vi "PreK12Login.vi"(2 "error in (no error)":errorcluster, 3 "Admin?":bool) -> (0 "error out":errorcluster, 1 "connection ID out":refnum<k5>)   [LabVIEW 2012]
uses:
  <userlib>/BotSpeak/Devices/EvalRIO/FTPCodes/FTPGlobals.vi
panel:
  out "passwrd":bool
  out "user":bool
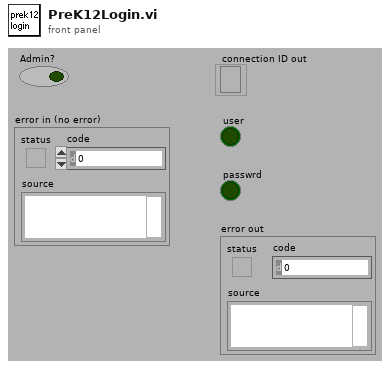
[diagram p1: front panel]
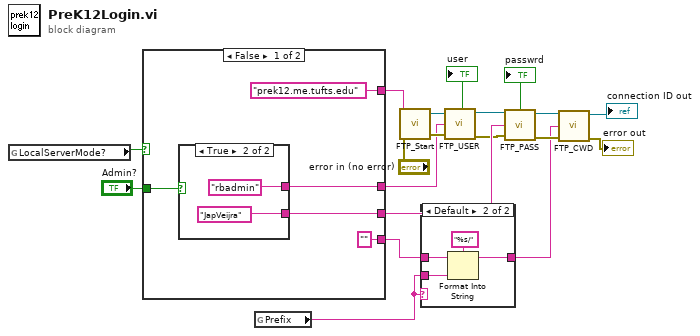
[diagram p0: block diagram]
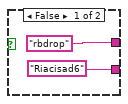
[diagram p3: hidden frame]
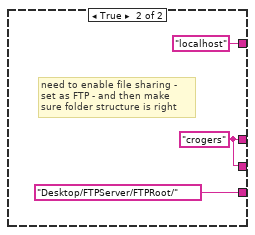
[diagram p4: hidden frame]
diagram:
  n1 = global read "FTPGlobals.vi" "LocalServerMode?"() -> (w2:bool)
  n2 = case shown="False" w2 {
    tunnel: [w24 w29] -> w14
    tunnel: [w23 w29] -> w13
    tunnel: "Admin?" -> [w22 _]
    tunnel: ["prek12.me.tufts.edu" ("address") "localhost" ("address")] -> w9
    tunnel: ["" ("password") "Desktop/FTPServer/FTPRoot/" ("password")] -> w4
    frame False {
      n3 = case shown="True" w22 {
        tunnel: ["rbdrop" ("user") "rbadmin" ("user")] -> w24
        tunnel: ["Riacisad6" ("password") "JapVeijra" ("password")] -> w23
        frame False {
        }
        frame True {
        }
      }
    }
    frame True {
      w29 = "crogers" ("user")
      # "need to enable file sharing - \nset as FTP - and then make\nsure folder structure is right"
    }
  }
  n4 = global read "FTPGlobals.vi" "Prefix"() -> (w1:string)
  n5 = call <userlib>:"FTP_Start.vi"("address"=w9, "error in (no error)"="error in (no error)") -> ("connection ID"=w16:refnum<k5>, "error out"=w15:errorcluster)  [unwired: 2 in, 2 out]
  n6 = case shown="Default" w1 {
    tunnel: w4 -> [w32 w36]
    tunnel: [w32 w34] -> w3
    tunnel: w1 -> [_ w33]
    frame "" {
    }
    frame Default {
      n7 = Format Into String(format string="%s/", initial string=w36, w33) -> (resulting string=w34:string)  [unwired: 1 in, 1 out]
    }
  }
  n8 = call <userlib>:"FTP_USER.vi"("connection ID"=w16, "user"=w14, "error out"=w15) -> ("connection ID out"=w10:refnum<k5>, "Good Reply?"=→"user":bool, "error out 2"=w11:errorcluster)  [unwired: 1 out]
  n9 = call <userlib>:"FTP_PASS.vi"("connection ID"=w10, "password"=w13, "error in"=w11) -> ("connection ID out"=w8:refnum<k5>, "Good Reply?"=→"passwrd":bool, "error out"=w7:errorcluster)  [unwired: 1 out]
  n10 = call <userlib>:"FTP_CWD.vi"("connection ID"=w8, "path"=w3, "error in"=w7) -> ("connection ID out"=→"connection ID out":refnum<k5>, "error out"=→"error out":errorcluster)  [unwired: 2 out]
